vi "PH_Beckhoff-16BB.panel.vi"(0 "object ref":refnum<vi>, 5 "error in (no error)":errorcluster) -> (19 "error out":errorcluster)   [LabVIEW 2014, in "PH_Beckhoff-16BB.lvlib"]
doc: "This a GUI.\n\nLicense Agreement for this software:\n\nCopyright (C)\nGesellschaft für Schwerionenforschung, GSI\nPlanckstr. 1\n64291 Darmstadt\nGermany\n\nContact: D.Beck@gsi.de \n\nThis program is free software; you can redistribute it and/or modify it under the terms of the GNU General Public License as published by the Free Software Foundation; either version 2 of the license, or (at your option) any later version.\n\nThis program is distributed in the hope that it will be useful, but WITHOUT ANYW ARRANTY; without even the implied warranty of MERCHANTABILITY or FITNESS FOR A PARTICULAR PURPOSE. See the GNU General License for more details (http://www.gnu.org).\n\nGesellschaft für Schwerionenforschung, GSI\nPlanckstr. 1, 64291 Darmstadt, Germany\nFor all questions and ideas contact: M.Richter@gsi.de, H.Brand@gsi.de or D.Beck@gsi.de.\nLast update: 18-DEC-2002"
uses:
  PH_Beckhoff-16BB.lvlib
  PH_Beckhoff/PH_Beckhoff.Connectivity.ctl
  PH_Beckhoff/PH_Beckhoff.ADS Error.ctl
  PH_Beckhoff/PH_Beckhoff.Values.ctl
  PH_Beckhoff/PH_Beckhoff.Sonderklemmen Inputs.ctl
  PH_Beckhoff/PH_Beckhoff.Analog Inputs.ctl
  PH_Beckhoff/PH_Beckhoff.Scaling Type.ctl
  PH_Beckhoff/PH_Beckhoff.Analog Outputs.ctl
  PH_Beckhoff/PH_Beckhoff.Digital Inputs.ctl
  PH_Beckhoff/PH_Beckhoff.Digital Outputs.ctl
  PH_Basics/PH_StatusHandler/PH_StatusHandler.GUI element.ctl
  PH_Beckhoff/PH_Beckhoff.GUI Refs.ctl
  CS_Core/CSObj/CSObj.lvlib
  PH_Basics/PH_Common/PH_Common.lvlib
  PH_Beckhoff/PH_Beckhoff.lvlib
  CS_Core/CSSystem/CSSystemLib/CSSystemLib.lvlib
  PH_Basics/PH_Class/PH_Class.lvlib
  PH_Basics/PH_StatusHandler/PH_StatusHandler.lvlib
panel:
  in  "Tab Control":enum32{"Beckhoff Stuff", "PA Chiller"}(tab)
  out "IP":string
  out "Connection":T1
  out "Prdc Int [ms]":i32
  out "Racktype":string
  out "ADS Error":T2
  out "Current Values":T3
  in  "Show Info":bool
  out "configured?":bool
  out "Chiller PSDB Status":u32(colorbox)=6618880 caption="PSDB"
  out "PA Chiller":T11={"_Status"=0, "Flow-control"=16860, "High-temp"=16860, "Conductivity"=16860, "Niveau"=16860}
  in  "Delete":bool
  in  "Exit":bool
  # "PCS"
  # "3.40"
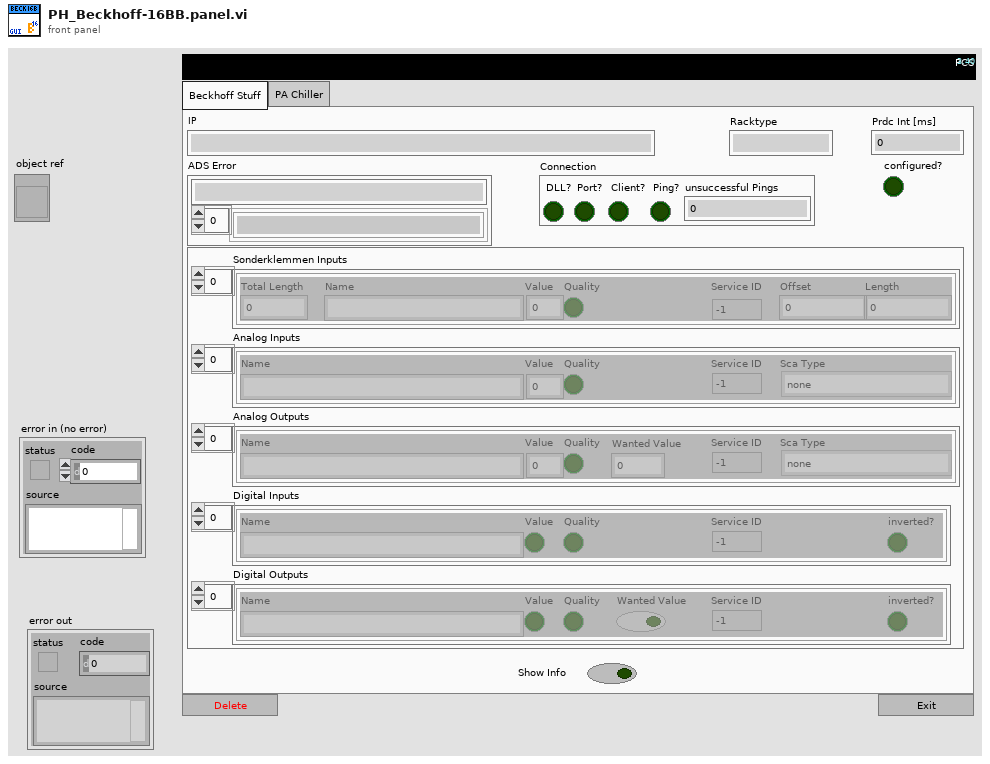
[diagram p1: front panel]
types:
  T1 = typedef "PH_Beckhoff.lvlib/PH_Beckhoff.Connectivity.ctl" = cluster{"DLL?":bool, "Port?":bool, "Client?":bool, "Ping?":bool, "unsuccessful Pings":u32}
  T2 = typedef "PH_Beckhoff.lvlib/PH_Beckhoff.ADS Error.ctl" = cluster{"Latest Error":string, "Error List":string[]}
  T3 = typedef "PH_Beckhoff.lvlib/PH_Beckhoff.Values.ctl" = cluster{"Sonderklemmen Inputs":T4, "Analog Inputs":T5, "Analog Outputs":T7, "Digital Inputs":T8, "Digital Outputs":T9}
  T4 = typedef "PH_Beckhoff.lvlib/PH_Beckhoff.Sonderklemmen Inputs.ctl" = cluster{"Total Length":u32, "Name":string, "Value":u64, "Quality":bool, "Service ID":i32, "Offset":u32, "Length":u32}[]
  T5 = typedef "PH_Beckhoff.lvlib/PH_Beckhoff.Analog Inputs.ctl" = cluster{"Name":string, "Value":u32, "Quality":bool, "Service ID":i32, "Sca Type":T6}[]
  T6 = typedef "PH_Beckhoff.lvlib/PH_Beckhoff.Scaling Type.ctl" = enum16{"none", "0 ... 15 Bit -> 0 ... 5", "0 ... 15 Bit -> 0 ... 10", "0 ... 15 Bit -> 0 ... 25", "0 ... 15 Bit -> 4 ... 20", "0 ... 15 Bit -> 0 ... 1", "0 ... 15 Bit -> 0 ... 20000", "0 ... 15 Bit -> 0 ... 24000"}
  T7 = typedef "PH_Beckhoff.lvlib/PH_Beckhoff.Analog Outputs.ctl" = cluster{"Name":string, "Value":u32, "Quality":bool, "Wanted Value":u32, "Service ID":i32, "Sca Type":T6}[]
  T8 = typedef "PH_Beckhoff.lvlib/PH_Beckhoff.Digital Inputs.ctl" = cluster{"Name":string, "Value":bool, "Quality":bool, "Service ID":i32, "inverted?":bool}[]
  T9 = typedef "PH_Beckhoff.lvlib/PH_Beckhoff.Digital Outputs.ctl" = cluster{"Name":string, "Value":bool, "Quality":bool, "Wanted Value":bool, "Service ID":i32, "inverted?":bool}[]
  T10 = typedef "PH_StatusHandler.lvlib/PH_StatusHandler.GUI element.ctl" = u16
  T11 = cluster{"_Status":T10, "Flow-control":u32, "High-temp":u32, "Conductivity":u32, "Niveau":u32}
  T12 = typedef "PH_Beckhoff.lvlib/PH_Beckhoff.GUI Refs.ctl" = cluster{"ADS Error":refnum<vi>, "Values":refnum<vi>, "configured?":refnum<vi>, "Connection":refnum<vi>, "IP":refnum<vi>, "Prdc Int [ms]":refnum<vi>}
  T13 = typedef "PH_Beckhoff.lvlib/PH_Beckhoff.i attribute.ctl" = cluster{"GUI Refs":T12, "operation?":bool, "Default Prdc Interval":i32, "Connection":T1, "AMS Net ID":T14, "Klemmencluster: # of":T15, "Values":T3, "IP":string, "Description":string, "configured?":bool, "Change Manager":cluster{"Detemination wanted?":bool, "Values changed at":cluster{"Sonderklemmen Inputs":i32[], "Analog Inputs":i32[], "Analog Outputs":i32[], "Digital Inputs":i32[], "Digital Outputs":i32[]}}, "Difference to handle an analog input as change":u32}
  T14 = typedef "Beckhoff - Driver np.lvlib/Beckhoff Access.ctl" = cluster{"DLL path":path, "AMS Net ID":cluster{"1st # of IP":u8, "2nd # of IP":u8, "3rd # of IP":u8, "4th # of IP":u8, "In Port":u8, "Out Port":u8}}
  T15 = typedef "Beckhoff - Driver np.lvlib/Klemmendeclarer.ctl" = cluster{"Offset due to Sonderklemms":u32, "analog Inputs":u32, "analog Outputs":u32, "digital Input Bits":u32, "digital Output Bits":u32}
  T16 = typedef "PH_Beckhoff-16BB.lvlib/PH_Beckhoff-16BB.i attribute.ctl" = cluster{"PA Chiller":cluster{"PSDB":cluster{"Status Service ID":i32, "Instance ID":i32, "Data Status":T17, "Ref Status":refnum<vi>, "Error Code":i32}, "Status":cluster{"GUI Ref":refnum<vi>, "Status Service ID":i32, "Status":T18}, "DIs":cluster{"Flow Control":cluster{"GUI Ref":refnum<vi>, "# in Data":i32}, "High-Temp":cluster{"GUI Ref":refnum<vi>, "# in Data":i32}, "Conductivity":cluster{"GUI Ref":refnum<vi>, "# in Data":i32}, "Niveau":cluster{"GUI Ref":refnum<vi>, "# in Data":i32}}, "PSDB Thread":cluster{"Ref":refnum<vi>, "Q-Ref":refnum<queue>}}, "PSDB":cluster{"Shot #":i32, "Subsystem":T19}, "Racktype":string, "PSDB Credentials":T20}
  T17 = typedef "PH_PSDBWriter.lvlib/PH_PSDBWriter.Data Status.ctl" = i16
  T18 = typedef "PH_StatusHandler.lvlib/PH_StatusHandler.Status.ctl" = i16
  T19 = typedef "PH_PSDBWriter.lvlib/PH_PSDBWriter.PHELIX-Subsystems.ctl" = i32
  T20 = typedef "PH_Common.lvlib/PH_Connection.PSDB Credentials.ctl" = cluster{"PW":string, "ID":string, "DS":string}
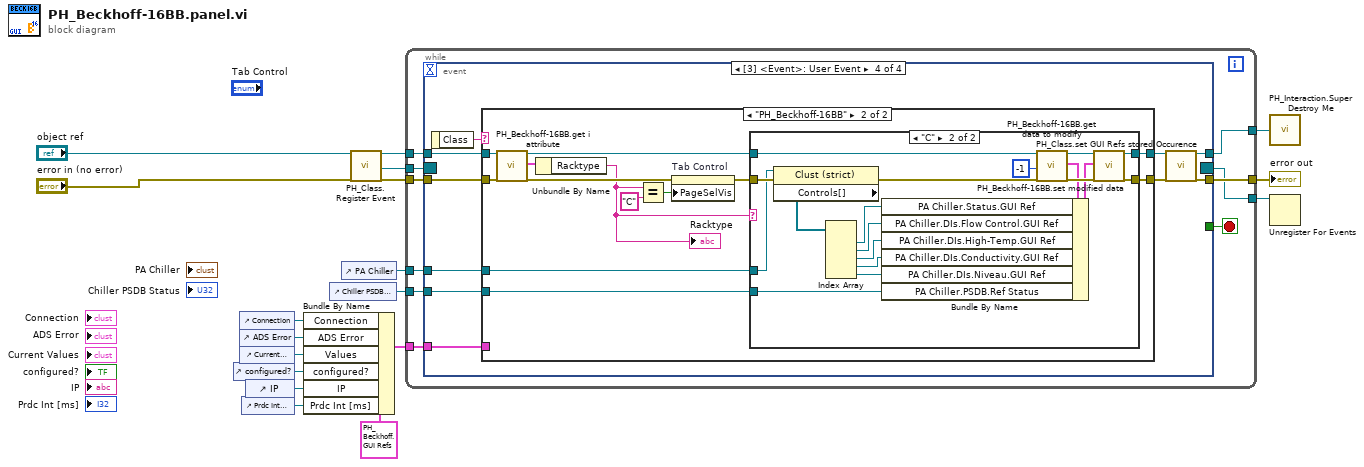
[diagram p0: block diagram]
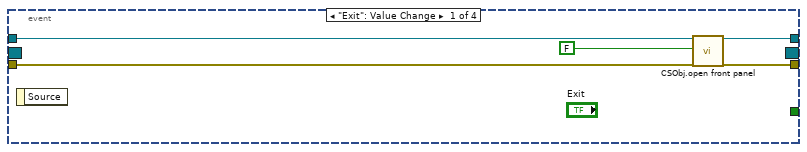
[diagram p2: hidden frame]
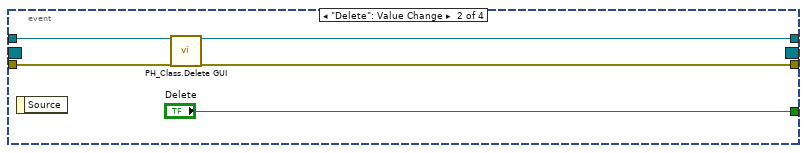
[diagram p3: hidden frame]
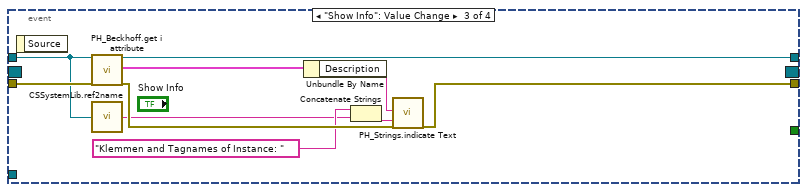
[diagram p4: hidden frame]
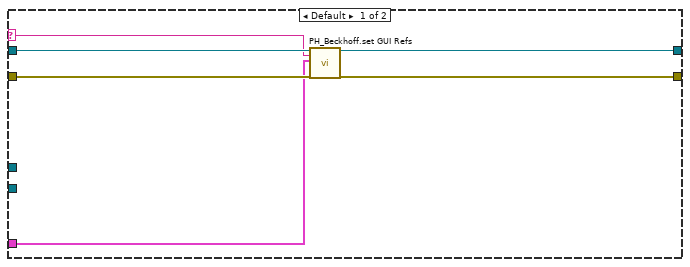
[diagram p5: hidden frame]
diagram:
  n1 = control-ref of="configured?"() -> (w12:refnum<vi>)
  n2 = control-ref of="Connection"() -> (w16:refnum<vi>)
  n3 = control-ref of="ADS Error"() -> (w15:refnum<vi>)
  n4 = control-ref of="Current Values"() -> (w13:refnum<vi>)
  n5 = control-ref of="Prdc Int [ms]"() -> (w3:refnum<vi>)
  n6 = control-ref of="IP"() -> (w4:refnum<vi>)
  n7 = Bundle By Name(cluster=T12 {"ADS Error"=refnum, "Values"=refnum, "configured?"=refnum, "Connection"=refnum, "IP"=refnum, "Prdc Int [ms]"=refnum} ("GUI Refs"), "Connection"=w16, "ADS Error"=w15, "Values"=w13, "configured?"=w12, "IP"=w4, "Prdc Int [ms]"=w3) -> (w5:T12)
  n8 = control-ref of="Chiller PSDB Status"() -> (w7:refnum<vi>)
  n9 = control-ref of="PA Chiller"() -> (w6:refnum<vi>)
  n10 = call "PH_Class.Register Event.vi"("i ref in"="object ref", "error in (no error)"="error in (no error)") -> ("i ref out"=w11:refnum<vi>, "Event Registration Refnum"=w9:refnum<event-registration>, "error out"=w10:errorcluster)  [unwired: 15 in]
  n11 = while {
    tunnel: w11 -> [w25]
    tunnel: [w24] -> w18
    tunnel: w10 -> [w27]
    tunnel: [w26] -> w17
    tunnel: w9 -> [w23]
    tunnel: [w22] -> w8
    tunnel: w7 -> [w21]
    tunnel: w6 -> [w20]
    tunnel: w5 -> [w19]
    stop <- w28 stop-if-true
    n12 = event shown="[3] <Event>: User Event" {
      selector: w23 -> [_ _ _ _]
      dyn-events: [_ _ _ _] -> w22
      timeout: _ -> [_ _ _ _]
      tunnel: [_ "Delete" _ _] -> w28
      tunnel: w25 -> [w30 w35 w39 w58]
      tunnel: w27 -> [w33 w37 w48 w57]
      tunnel: [w32 w36 w45 w51] -> w26
      tunnel: [w29 w34 w47 w49] -> w24
      tunnel: w21 -> [_ _ _ w54]
      tunnel: w20 -> [_ _ _ w53]
      tunnel: w19 -> [_ _ _ w52]
      event "Exit": Value Change {
        n13 = event-data() -> ()  [unwired: 1 in, 1 out]
        n14 = call "CSObj.open front panel.vi"("i ref in"=w30, "frontPanelOpen"=FALSE ("front panel open"), "error in (no error)"=w33) -> ("i ref out"=w29:refnum<vi>, "error out"=w32:errorcluster)  [unwired: 15 in]
      }
      event "Delete": Value Change {
        n15 = event-data() -> ()  [unwired: 1 in, 1 out]
        n16 = call "PH_Class.Delete GUI.vi"("VI in"=w35, "error in (no error)"=w37) -> ("VI out"=w34:refnum<vi>, "error out"=w36:errorcluster)  [unwired: 16 in]
      }
      event "Show Info": Value Change {
        n17 = event-data() -> ()  [unwired: 1 in, 1 out]
        n18 = call "PH_Beckhoff.get i attribute.vi"("i ref in"=w39, "error in (no error)"=w48) -> ("i ref out"=w47:refnum<vi>, "i attribute"=w44:T13, "error out"=w46:errorcluster)  [unwired: 15 in]
        n19 = call "CSSystemLib.ref2name.vi"("obj refnum"=w39) -> ("name"=w40:string)
        n20 = Unbundle By Name(w44) -> ("Description"=w43:string)
        n21 = Concatenate Strings("Klemmen and Tagnames of Instance: " ("Caption.Text"), w40) -> (w41:string)
        n22 = call "PH_Strings.indicate Text.vi"("String to show"=w43, "Caption.Text"=w41, "error in (no error)"=w46) -> ("error out"=w45:errorcluster)  [unwired: 16 in]
      }
      event User Event {
        n23 = event-data() -> ("Class"=w55:string)  [unwired: 1 in]
        n24 = case shown="\"PH_Beckhoff-16BB\"" w55 {
          selector: w55 -> [w60 _]
          tunnel: w58 -> [w64 w72]
          tunnel: w57 -> [w62 w77]
          tunnel: [w63 w76] -> w50
          tunnel: [w61 w75] -> w56
          tunnel: w54 -> [_ w74]
          tunnel: w53 -> [_ w73]
          tunnel: w52 -> [w59 _]
          frame Default {
            n25 = call "PH_Beckhoff.set GUI Refs.vi"("i ref in"=w64, "Class"=w60, "GUI Refs"=w59, "error in"=w62) -> ("i ref out"=w63:refnum<vi>, "error out"=w61:errorcluster)  [unwired: 14 in]
          }
          frame "PH_Beckhoff-16BB" {
            n26 = call "PH_Beckhoff-16BB.get i attribute.vi"("i ref in"=w72, "error in (no error)"=w77) -> ("i ref out"=w71:refnum<vi>, "i attribute"=w70:T16, "error out"=w69:errorcluster)  [unwired: 15 in]
            n27 = Unbundle By Name(w70) -> ("Racktype"=w66:string)
            "Racktype" <- w66
            n28 = Equal?(x=w66, y="C") -> (x = y?=w65:bool)
            n29 = property on="Tab Control" class="TabCtl (strict)"(error in=w69, "PageSelVis"=w65) -> (error out=w68:errorcluster)  [unwired: 1 in, 1 out]
            n30 = case shown="\"C\"" w66 {
              tunnel: w68 -> [w78 w91]
              tunnel: [w78 w81] -> w75
              tunnel: w71 -> [w79 w96]
              tunnel: [w79 w82] -> w76
              tunnel: w73 -> [_ w88]
              tunnel: w74 -> [_ w92]
              frame Default {
              }
              frame "C" {
                n31 = property class="Clust (strict)"(reference=w88, error in=w91) -> (error out=w90:errorcluster, "Controls[]"=w89:refnum<vi>[])  [unwired: 1 out]
                n32 = Index Array(array=w89) -> (element #1=w87:refnum<vi>, element #2=w86:refnum<vi>, element #3=w85:refnum<vi>, element #4=w84:refnum<vi>, element #5=w83:refnum<vi>)  [unwired: 5 in]
                n33 = call "PH_Beckhoff-16BB.get data to modify.vi"("i ref in"=w96, "ms timeout (10000)"=-1, "error in (no error)"=w90) -> ("i ref out"=w95:refnum<vi>, "i attribute"=w94:T16, "error out"=w97:errorcluster)  [unwired: 13 in, 1 out]
                n34 = Bundle By Name(cluster=w94, "PA Chiller.Status.GUI Ref"=w87, "PA Chiller.DIs.Flow Control.GUI Ref"=w86, "PA Chiller.DIs.High-Temp.GUI Ref"=w85, "PA Chiller.DIs.Conductivity.GUI Ref"=w84, "PA Chiller.DIs.Niveau.GUI Ref"=w83, "PA Chiller.PSDB.Ref Status"=w92) -> (w80:T16)
                n35 = call "PH_Beckhoff-16BB.set modified data.vi"("i ref in"=w95, "i attribute"=w80, "error in (no error)"=w97) -> ("i ref out"=w82:refnum<vi>, "error out"=w81:errorcluster)  [unwired: 15 in]
              }
            }
          }
        }
        n36 = call "PH_Class.set GUI Refs stored Occurence.vi"("i ref in"=w50, "error in (no error)"=w56) -> ("i ref out"=w49:refnum<vi>, "error out"=w51:errorcluster)  [unwired: 16 in]
      }
    }
  }
  "error out" <- w17
  n37 = call "PH_Interaction.Super Destroy Me.vi"("i ref out"=w18) -> ()
  n38 = Unregister For Events(event registration refnum=w8) -> ()  [unwired: 1 in, 1 out]
